vi "fgv_ctrl-refs_old3.vi"(7 "cmd":enum16{"read", "write"}(ring), 11 "ctrl ref":refnum<vi>[](array[refnum])) -> (3 "ctrl ref out":refnum<vi>[](array[refnum]))   [LabVIEW 2019]
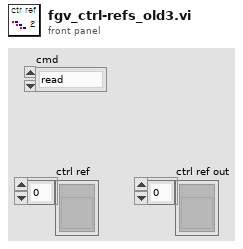
[diagram p1: front panel]
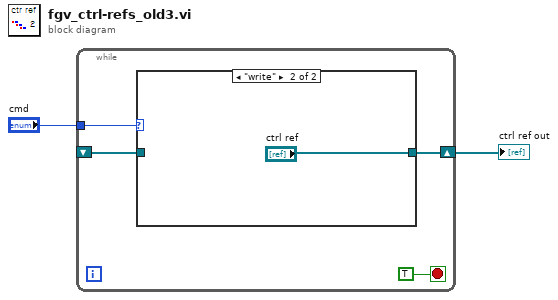
[diagram p0: block diagram]
diagram:
  n1 = while {
    tunnel: "cmd" -> [w5]
    shift-right: [w4] -> w1
    shift-left: _ -> [w3]
    stop <- TRUE stop-if-true
    n2 = case shown="\"write\"" w5 {
      tunnel: [w7 "ctrl ref"] -> w4
      tunnel: w3 -> [w7 _]
      frame "read", Default {
      }
      frame "write" {
      }
    }
  }
  "ctrl ref out" <- w1
